vi "CalculateFps.vi"(11 "New Frames Transferred":u64) -> (3 "Frames/s":dbl)   [LabVIEW 2021]
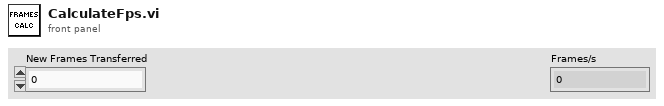
[diagram p1: front panel]
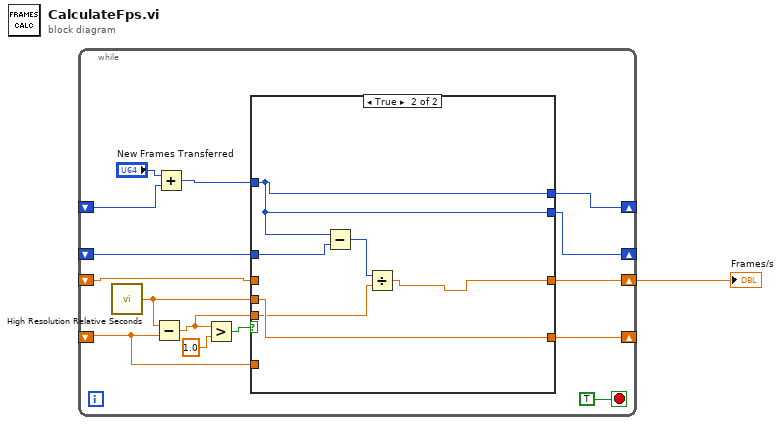
[diagram p0: block diagram]
diagram:
  n1 = while {
    shift-right: [w6] -> _
    shift-left: _ -> [w14]
    shift-right: [w12] -> _
    shift-left: _ -> [w11]
    shift-right: [w8] -> w1
    shift-left: _ -> [w7]
    shift-right: [w2] -> _
    shift-left: _ -> [w3]
    stop <- TRUE stop-if-true
    n2 = call <vilib>:"High Resolution Relative Seconds.vi"() -> ("relative seconds"=w13:dbl)
    n3 = Subtract(x=w13, y=w11) -> (x-y=w10:dbl)
    n4 = Add(x="New Frames Transferred", y=w3) -> (x+y=w4:u64)
    n5 = Greater?(x=w10, y=1.0) -> (0:w15:bool)
    n6 = case shown="True" w15 {
      tunnel: w14 -> [w20 w26]
      tunnel: [w20 w21] -> w6
      tunnel: w13 -> [_ w25]
      tunnel: [w19 w25] -> w12
      tunnel: w11 -> [w19 _]
      tunnel: w10 -> [_ w23]
      tunnel: [w18 w22] -> w8
      tunnel: w7 -> [w18 _]
      tunnel: w4 -> [w17 w21]
      tunnel: [w17 w21] -> w2
      frame False {
      }
      frame True {
        n7 = Subtract(x=w21, y=w26) -> (x-y=w24:u64)
        n8 = Divide(x=w24, y=w23) -> (x/y=w22:dbl)
      }
    }
  }
  "Frames/s" <- w1
